vi "fft_filtering.vi"(6 "Noise limit":bool, 7 "Reset":bool, 9 "Data":dbl[](array[numeric]), 10 "Config":T2={"I/O"={"Buffering (in/out)"=[], "Output Device"=0, "Sound"={"sample rate (S/s)"=0.0, "number of channels"=0, "bits per sample"=0}, "Input Device"=0}, "Noise limit low"=0.0, "Distortion LF cut"=0.0, "Averaging Tc"=0.0, "High rate STFT"={"Win param"=101.5, "Window type"=61, "Win order"=2, "DFT size"=64, "Channels"=[7], "Oversample"=64}, "Low rate STFT"={"Win param"=120.0, "Window type"=61, "Win order"=8, "DFT size"=64, "Channels"=[7], "Oversample"=64}, "Hum filter"={"Frequency"=0.0, "Tc"=0.0}} {"Low rate STFT"."Oversample" min=1 step=1; "Low rate STFT"."Channels" min=0 step=1; "Low rate STFT"."DFT size" min=1 step=1; "Low rate STFT"."Window type" items=["Rectangle"=0, "Hanning"=1, "Hamming"=2, "Blackman-Harris"=3, "Exact Blackman"=4, "Blackman"=5, "Flat Top"=6, "4 Term B-Harris "=7, "7 Term B-Harris"=8, "Low Sidelobe"=9, "Blackman Nuttall"=11, "Triangle"=30, "Bartlett-Hanning"=31, "Bohman"=32, "Parzen"=33, "Welch"=34, "Kaiser"=60, "Dolph-Chebyshev"=61, "Gaussian"=62]; "High rate STFT"."Oversample" min=1 step=1; "High rate STFT"."Channels" min=0 step=1; "High rate STFT"."DFT size" min=1 step=1; "High rate STFT"."Window type" items=["Rectangle"=0, "Hanning"=1, "Hamming"=2, "Blackman-Harris"=3, "Exact Blackman"=4, "Blackman"=5, "Flat Top"=6, "4 Term B-Harris "=7, "7 Term B-Harris"=8, "Low Sidelobe"=9, "Blackman Nuttall"=11, "Triangle"=30, "Bartlett-Hanning"=31, "Bohman"=32, "Parzen"=33, "Welch"=34, "Kaiser"=60, "Dolph-Chebyshev"=61, "Gaussian"=62]; "I/O"."Input Device" format="%.0x"; "I/O"."Output Device" format="%.0x"}, 11 "Modulation info":T1 {"Hi channels at low" min=0 step=1; "Low carriers" format="%#_6p"; "High carriers" format="%#_6p"}) -> (1 "Carrier model":dbl[](array[numeric]), 2 "Distortion model":dbl[](array[numeric]), 3 "Averaged FFT":cdb[](array[numeric]))   [LabVIEW 2014]
uses:
  ilemt_config.ctl
  <vilib>/sound2/lvsound2.llb/Sound Data Format.ctl
  stft_params.ctl
  <vilib>/Analysis/4window.llb/windowTd.ctl
  modulation_info.ctl
  <vilib>/Analysis/2dsp.llb/Real FFT.vi
  <vilib>/Analysis/2dsp.llb/Inverse Real FFT.vi
  <vilib>/Analysis/NI_AALPro.lvlib
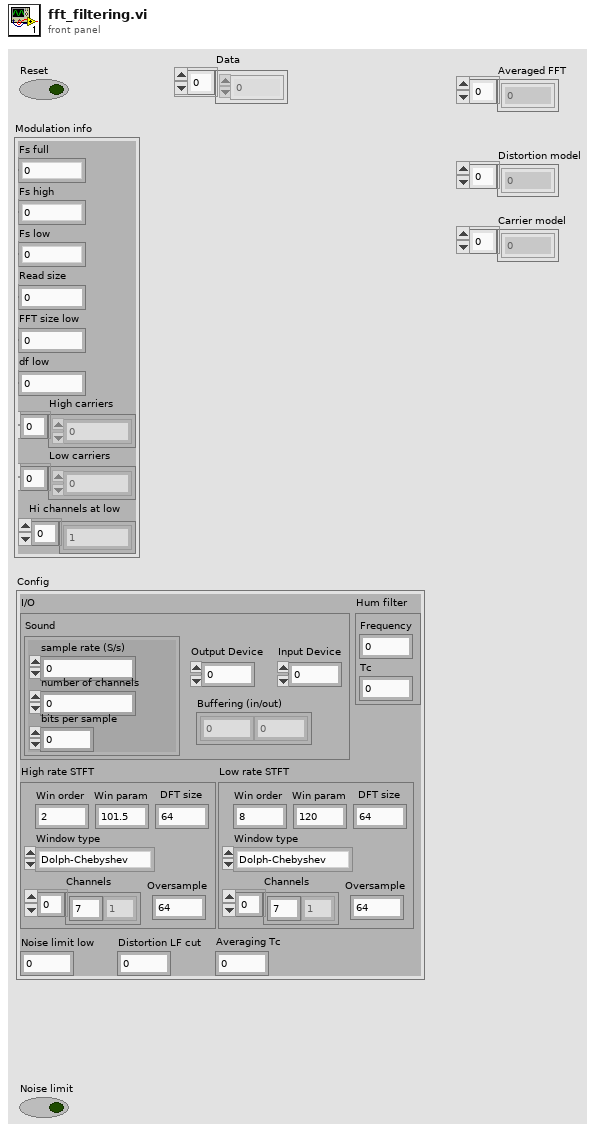
[diagram p1: front panel]
types:
  T1 = typedef "modulation_info.ctl" = cluster{"Fs full":dbl, "Fs high":dbl, "Fs low":dbl, "Read size":i32, "FFT size low":i32, "df low":dbl, "High carriers":dbl[], "Low carriers":dbl[], "Hi channels at low":i32[]}
  T2 = typedef "ilemt_config.ctl" = cluster{"I/O":cluster{"Buffering (in/out)":dbl[], "Output Device":u32, "Sound":T3, "Input Device":u32}, "Noise limit low":dbl, "Distortion LF cut":dbl, "Averaging Tc":sgl, "High rate STFT":T4, "Low rate STFT":T4, "Hum filter":cluster{"Frequency":dbl, "Tc":dbl}}
  T3 = typedef "Sound Data Format.ctl" = cluster{"sample rate (S/s)":dbl, "number of channels":i32, "bits per sample":i32}
  T4 = typedef "stft_params.ctl" = cluster{"Win param":dbl, "Window type":T5, "Win order":i32, "DFT size":i32, "Channels":i32[], "Oversample":i32}
  T5 = typedef "NI_AALPro.lvlib/windowTd.ctl" = u32
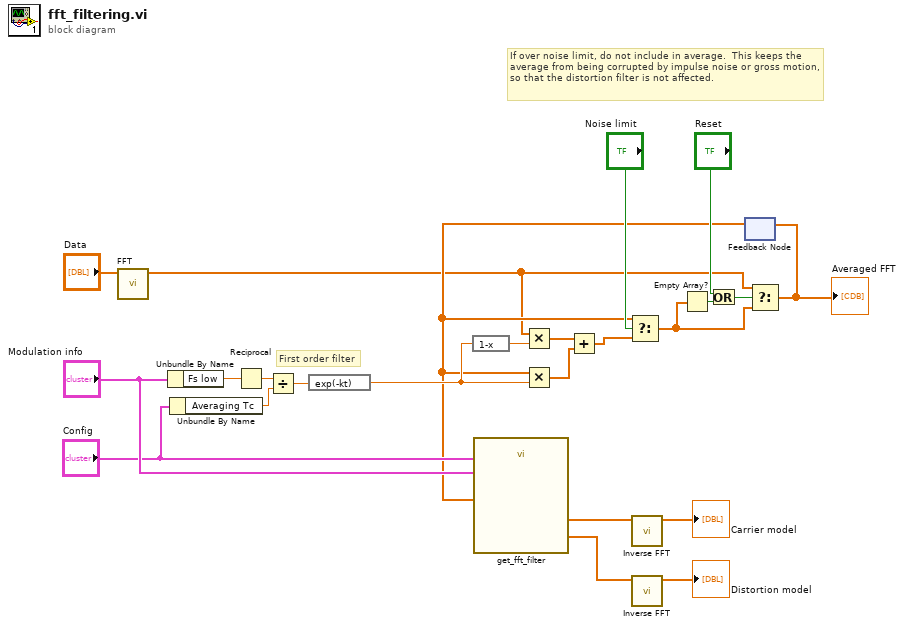
[diagram p0: block diagram]
diagram:
  # "If over noise limit, do not include in average.  This keeps the average from being corrupted by impulse noise or gross motion, so that the distortion filter is not affected."
  # "First order filter"
  n1 = call-poly <vilib>:"FFT.vi"("X"="Data") -> ("FFT {X}"=w5:cdb[])  [unwired: 9 in, 1 out]
  n2 = Unbundle By Name("Modulation info") -> ("Fs low"=w13:dbl)
  n3 = Unbundle By Name("Config") -> ("Averaging Tc"=w24:sgl)
  n4 = Reciprocal(x=w13) -> (1/x=w12:dbl)
  n5 = Divide(x=w12, y=w24) -> (x/y=w17:dbl)
  n6 = expression code="exp(-kt)"(w17) -> (w15:dbl)
  n7 = expression code="1-x"(w15) -> (w16:dbl)
  n8 = Multiply(x=w5, y=w16) -> (x*y=w14:cdb[])
  n9 = feedback #1() -> (w7:cdb[])  [unwired: 1 in]
  n10 = call "get_fft_filter.vi"("Modulation info"="Modulation info", "Config"="Config", "Averaged FFT"=w7) -> ("Carrier model"=w4:cdb[], "Distortion filter"=w1:cdb[])  [unwired: 7 in]
  n11 = Multiply(x=w7, y=w15) -> (x*y=w9:cdb[])
  n12 = Add(x=w14, y=w9) -> (x+y=w18:cdb[])
  n13 = Select(t=w7, s="Noise limit", f=w18) -> (s? t:f=w20:cdb[])
  n14 = call-poly <vilib>:"Inverse FFT.vi"("FFT {X}"=w4) -> ("X"=→"Carrier model":dbl[])  [unwired: 9 in, 1 out]
  n15 = call-poly <vilib>:"Inverse FFT.vi"("FFT {X}"=w1) -> ("X"=→"Distortion model":dbl[])  [unwired: 9 in, 1 out]
  n16 = Empty Array?(array=w20) -> (empty?=w21:bool)
  n17 = Or(x="Reset", y=w21) -> (x .or. y?=w23:bool)
  n18 = Select(t=w5, s=w23, f=w20) -> (s? t:f=w8:cdb[])
  "Averaged FFT" <- w8
  n19 = feedback-in #1(w8) -> ()
